vi "copySecFromIniToTable.vi"(10 "valInCol0":string) -> (2 "arrWithSec":string[](array[string]))   [LabVIEW 2010]
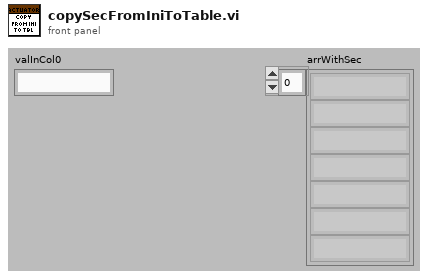
[diagram p1: front panel]
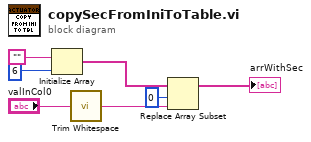
[diagram p0: block diagram]
diagram:
  n1 = Initialize Array("", 6 ("dimension size")) -> (w2:string[])
  n2 = call <vilib>:"Trim Whitespace.vi"("string"="valInCol0") -> ("trimmed string"=w5:string)  [unwired: 1 in]
  n3 = Replace Array Subset(array=w2, new element=w5, index=0) -> (→"arrWithSec":string[])
